vi "SP Read Single.vi"(8 "error in":errorcluster, 9 "Channel Index":i32=1, 11 "Humidity Setpoint in":refnum<class "Humidity Setpoint.lvclass">) -> (0 "error out":errorcluster, 1 "Changed or First Call?":bool, 2 "Humidity SP":dbl, 3 "Humidity Setpoint out":refnum<class "Humidity Setpoint.lvclass">)   [LabVIEW 2023, in "Humidity Setpoint.lvclass"]
uses:
  Humidity Setpoint.lvclass
  Parents/Setpoint/Setpoint.lvclass
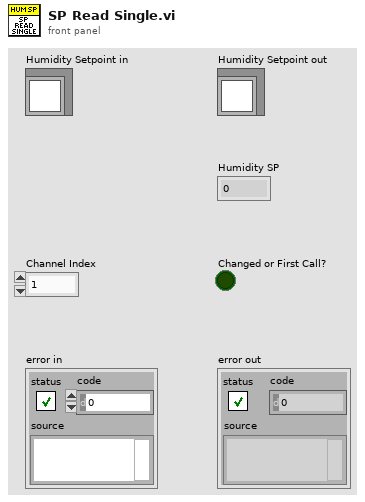
[diagram p1: front panel]
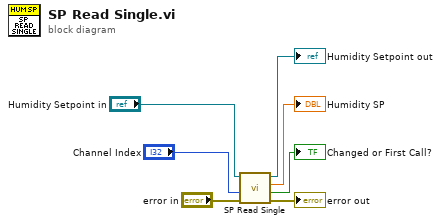
[diagram p0: block diagram]
diagram:
  n1 = call-parent "SP Read Single.vi"("error in"="error in", "Channel Index"="Channel Index", "Setpoint in"="Humidity Setpoint in") -> ("error out"=→"error out":errorcluster, "Changed or First Call?"=→"Changed or First Call?":bool, "Current SP"=→"Humidity SP":dbl, "Setpoint out"=→"Humidity Setpoint out":refnum<class "Humidity Setpoint.lvclass">)  [unwired: 5 in]
